vi "Create Message Group_ex.vi"() -> ()   [LabVIEW 2019]
uses:
  <vilib>/NI VeriStand/Custom Device API/Custom Device Item Ref.ctl
  Scripting API/Scripting API.lvlib
  <vilib>/NI VeriStand/Custom Device API/Custom Device API.lvlib
panel:
  out "Instrument Addon Refnum Out":T1=18446744073709551615 format="%.0x"
  out "Message Group Refnum":T1=18446744073709551615 format="%.0x"
  out "Error Out":errorcluster
  in  "Instrument Addon Refnum In":T1=18446744073709551615 format="%.0x"
  in  "Message Group Name":string
  in  "Error In":errorcluster
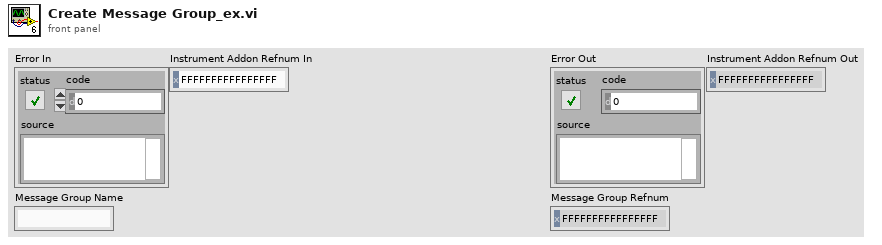
[diagram p1: front panel]
types:
  T1 = typedef "Custom Device API.lvlib/Custom Device Item Ref.ctl" = u64
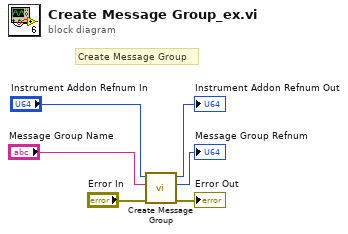
[diagram p0: block diagram]
diagram:
  # "Create Message Group"
  n1 = call "Create Message Group.vi"("Error In"="Error In", "Message Group Name"="Message Group Name", "Instrument Addon Refnum In"="Instrument Addon Refnum In") -> ("Error Out"=→"Error Out":errorcluster, "Message Group Refnum"=→"Message Group Refnum":T1, "Instrument Addon Refnum Out"=→"Instrument Addon Refnum Out":T1)  [unwired: 6 in]
